vi "Unregister Event(Customize Event and Register).vi"(8 "error in (no error)":errorcluster, 10 "Event Type":T1=enum."Initialize Finish", 11 "Register Name":string) -> (0 "error out":errorcluster)   [LabVIEW 2019, in "FootScan Engine Event.lvlib"]
uses:
  FootScan Engine Event.lvlib
  Event Type.ctl
  <userlib>/JUL/Event Message Module/Event Message Library/Event Action.ctl
panel:
  # "Input"
  # "Output"
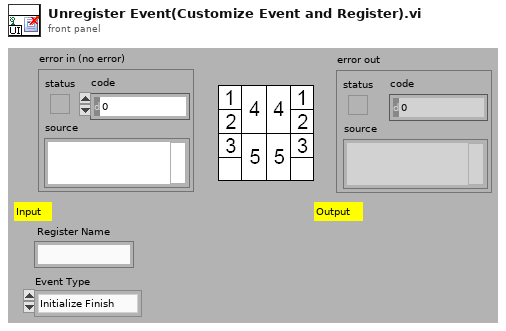
[diagram p1: front panel]
types:
  T1 = typedef "FootScan Engine Event.lvlib/Event Type.ctl" = enum16{"Default", "Initialize Finish", "Button 0 Click", "Exit Click", "Exit"}
  T2 = typedef "Event Action.ctl" = enum16{"Default", "Generate Event", "Register", "Unregister(Customize Event and Register)", "Unregister(All Events In Customize Register)", "Unregister(All Registers In Customize Event)", "Get Register Table"}
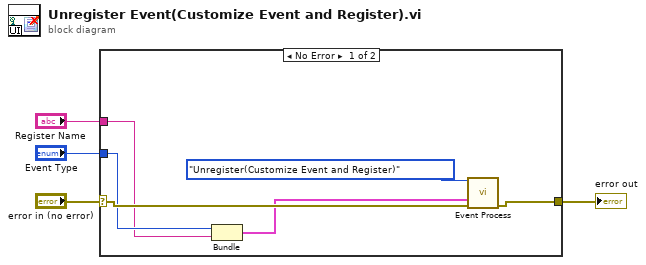
[diagram p0: block diagram]
diagram:
  n1 = case shown="No Error" "error in (no error)" {
    selector: "error in (no error)" -> [w9 w11]
    tunnel: [w10 w11] -> w1
    tunnel: "Event Type" -> [w7 _]
    tunnel: "Register Name" -> [w6 _]
    frame No Error {
      n2 = Bundle("Event Type"=w7, "Register Name"=w6) -> (w5:cluster{"Event Type":T1, "Register Name":string})  [unwired: 1 in]
      n3 = call "Event Process.vi"("Event Action"=Event_Action."Unregister(Customize Event and Register)", "Unregister Event Data(Customize Event and Register)"=w5, "error in (no error)"=w9) -> ("error out"=w10:errorcluster)  [unwired: 11 in, 1 out]
    }
    frame Error {
    }
  }
  "error out" <- w1
